vi "Write Camera Status.vi"(8 "error in (no error)":errorcluster, 10 "Camera Status":T1, 11 "Interface in":refnum<class "Interface.lvclass">) -> (0 "error out":errorcluster, 3 "Interface out":refnum<class "Interface.lvclass">)   [LabVIEW 2012, in "Interface.lvclass"]
uses:
  Interface.lvclass
  Interface.lvclass/Interface.ctl
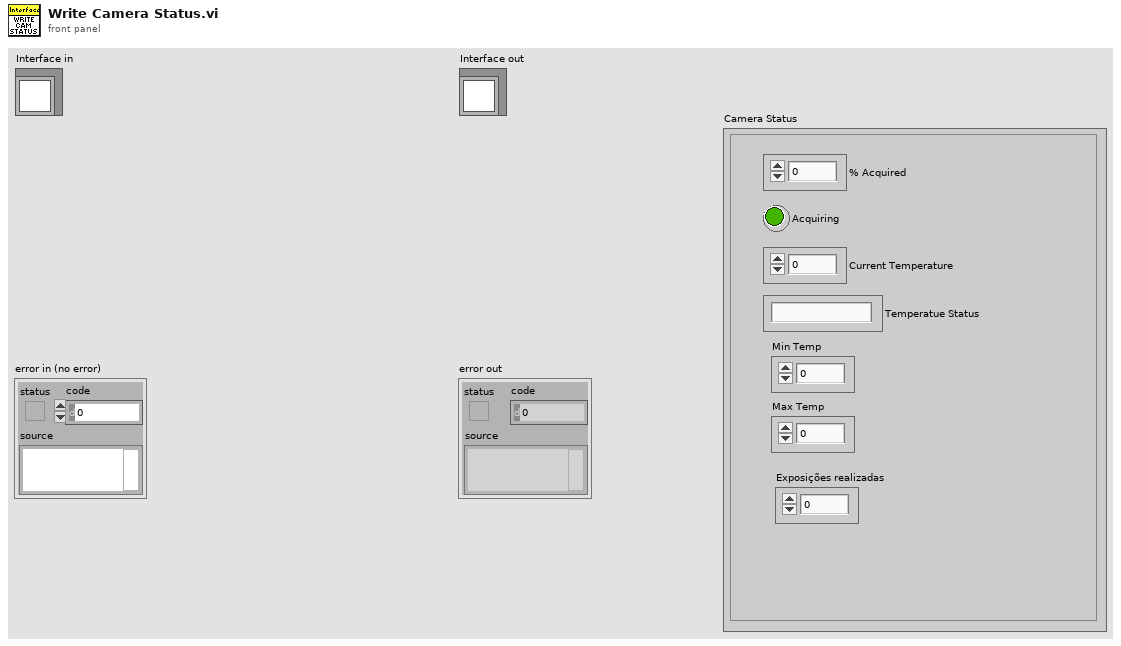
[diagram p1: front panel]
types:
  T1 = cluster{"% Acquired":dbl, "Acquiring":bool, "Current Temperature":dbl, "Temperatue Status":string, "Min Temp":dbl, "Max Temp":dbl, "Exposições realizadas":u32}
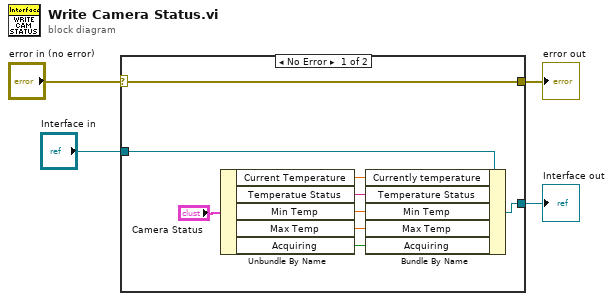
[diagram p0: block diagram]
diagram:
  n1 = case shown="No Error" "error in (no error)" {
    selector: "error in (no error)" -> [w13 w15]
    tunnel: [w13 w15] -> w3
    tunnel: [w11 w14] -> w1
    tunnel: "Interface in" -> [w12 w14]
    frame No Error {
      n2 = Unbundle By Name("Camera Status") -> ("Current Temperature"=w9:dbl, "Temperatue Status"=w10:string, "Min Temp"=w8:dbl, "Max Temp"=w7:dbl, "Acquiring"=w5:bool)
      n3 = Bundle By Name(cluster=w12, "Currently temperature"=w9, "Temperature Status"=w10, "Min Temp"=w8, "Max Temp"=w7, "Acquiring"=w5) -> (w11:refnum<class "Interface.lvclass">)
    }
    frame Error {
    }
  }
  "error out" <- w3
  "Interface out" <- w1
